vi "Get Class Name.vi"(1 "board in":refnum<class "Board Design.lvclass">) -> (0 "class name":string)   [LabVIEW 2023, in "Board Design.lvclass"]
doc: "Get the name of this class."
uses:
  Board Design.lvclass
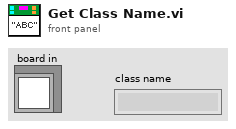
[diagram p1: front panel]
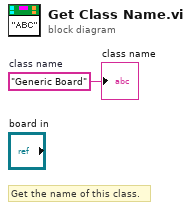
[diagram p0: block diagram]
diagram:
  w1 = "Generic Board"  # class name
  # "Get the name of this class."
  "class name" <- w1
